vi "Get Tx UDP All Channels.vi"(8 "error in":errorcluster, 11 "custom device ref in":T1 format="%.0x") -> (0 "error out":errorcluster, 2 "Tx UDP channel refs out":T1[](array[typedef]) format="%.0x", 3 "custom device ref out":T1 format="%.0x")   [LabVIEW 2020, in "AIM ARINC 664 Scripting.lvlib"]
uses:
  AIM ARINC 664 Scripting.lvlib
  <vilib>/NI VeriStand/Custom Device Tools/Custom Device Utility Library/Custom Device Utility Library.lvlib
  <vilib>/NI VeriStand/Custom Device API/Custom Device Item Ref.ctl
  <vilib>/NI VeriStand/Custom Device API/Custom Device API.lvlib
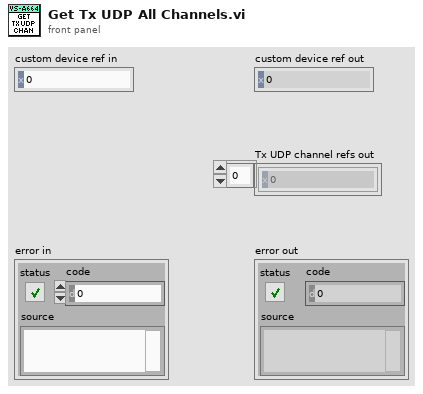
[diagram p1: front panel]
types:
  T1 = typedef "Custom Device API.lvlib/Custom Device Item Ref.ctl" = u64
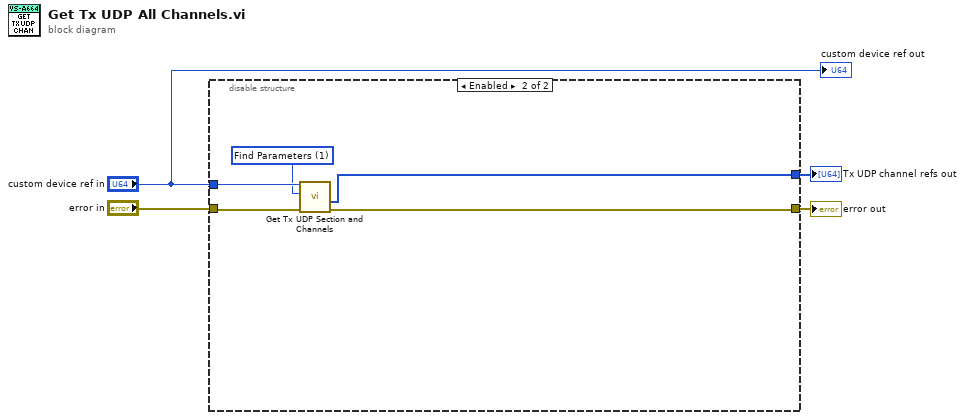
[diagram p0: block diagram]
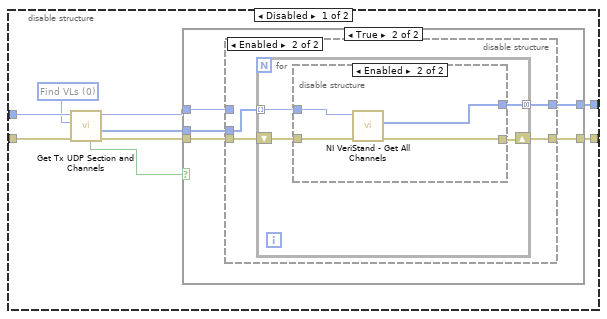
[diagram p2: hidden frame]
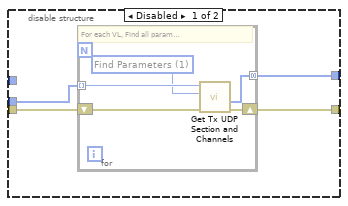
[diagram p4: hidden frame]
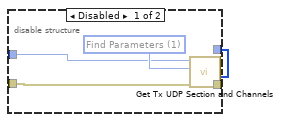
[diagram p5: hidden frame]
diagram:
  n1 = disable-structure shown="Enabled" {
    disable-tunnel: [w13 w47] -> w4
    disable-tunnel: [w11 w46] -> w3
    disable-tunnel: "error in" -> [w9 w49]
    disable-tunnel: "custom device ref in" -> [w7 w50]
    frame Disabled {
      w5 = u16 0 items=["Find VLs", "Find Parameters"] ("Option")
      n2 = call "Get Tx UDP Section and Channels.vi"("error in"=w9, "option"=w5, "custom device ref in"=w7) -> ("error out"=w12:errorcluster, "Tx UDP channel refs out"=w10:T1[], "custom device ref out"=w8:T1, "channels found?"=w6:bool)  [unwired: 3 in, 2 out]
      n3 = case shown="True" w6 {
        tunnel: [w14 w19] -> w13
        tunnel: w12 -> [w14 w18]
        tunnel: [_ w17] -> w11
        tunnel: w10 -> [_ w16]
        tunnel: w8 -> [_ w15]
        frame False {
        }
        frame True {
          n4 = disable-structure shown="Enabled" {
            disable-tunnel: [w23 w30] -> w19
            disable-tunnel: w18 -> [w22 w32]
            disable-tunnel: [w21 w29] -> w17
            disable-tunnel: w16 -> [w20 w31]
            disable-tunnel: w15 -> [_ _]
            frame Disabled {
              n5 = for {
                tunnel: w20 -> [w28] mode=indexing
                tunnel: [w26] -> w21 mode=concatenating
                shift-right: [w24] -> w23
                shift-left: w22 -> [w25]
                w27 = u16 1 items=["Find VLs", "Find Parameters"] ("Option")
                # "For each VL, Find all param Channels(parameters)"
                n6 = call "Get Tx UDP Section and Channels.vi"("error in"=w25, "option"=w27, "custom device ref in"=w28) -> ("error out"=w24:errorcluster, "Tx UDP channel refs out"=w26:T1[])  [unwired: 3 in, 4 out]
              }
            }
            frame Enabled {
              n7 = for {
                tunnel: w31 -> [w36] mode=indexing
                tunnel: [w35] -> w29 mode=concatenating
                shift-right: [w34] -> w30
                shift-left: w32 -> [w33]
                n8 = disable-structure shown="Enabled" {
                  disable-tunnel: w36 -> [w40 w44]
                  disable-tunnel: [w39 w43] -> w35
                  disable-tunnel: [w38 w42] -> w34
                  disable-tunnel: w33 -> [w37 w45]
                  frame Disabled {
                    w41 = u16 1 items=["Find VLs", "Find Parameters"] ("Option")
                    n9 = call "Get Tx UDP Section and Channels.vi"("error in"=w37, "option"=w41, "custom device ref in"=w40) -> ("error out"=w38:errorcluster, "Tx UDP channel refs out"=w39:T1[])  [unwired: 3 in, 4 out]
                  }
                  frame Enabled {
                    n10 = call <vilib>:"NI VeriStand - Get All Channels.vi"("error in"=w45, "Section Ref in"=w44) -> ("error out"=w42:errorcluster, "Channel Refs"=w43:T1[])  [unwired: 6 in, 2 out]
                  }
                }
              }
            }
          }
        }
      }
    }
    frame Enabled {
      w48 = u16 1 items=["Find VLs", "Find Parameters"] ("option")
      n11 = call "Get Tx UDP Section and Channels.vi"("error in"=w49, "option"=w48, "custom device ref in"=w50) -> ("error out"=w47:errorcluster, "Tx UDP channel refs out"=w46:T1[])  [unwired: 3 in, 4 out]
    }
  }
  "error out" <- w4
  "Tx UDP channel refs out" <- w3
  "custom device ref out" <- "custom device ref in"
